vi "Load App.vi"(8 "error in (no error)":errorcluster) -> (0 "error out":errorcluster)   [LabVIEW 2013, in "LVAutomationListener.lvlib" / "LVAutomationListener.lvclass"]
doc: "Load the application into memory and start it running. The input notifier is used to send text to the splash screen to tell the user what stage the load process is in."
uses:
  LVAutomationListener.lvclass
  <vilib>/ActorFramework/Message Queue/Message Queue.lvclass/Message Queue.ctl
  <vilib>/Utility/error.llb/DialogType.ctl
  <vilib>/ActorFramework/Actor/Actor.lvclass
  <vilib>/ActorFramework/Message Queue/Message Queue.lvclass
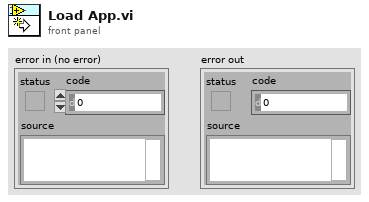
[diagram p1: front panel]
types:
  T1 = typedef "DialogType.ctl" = u16
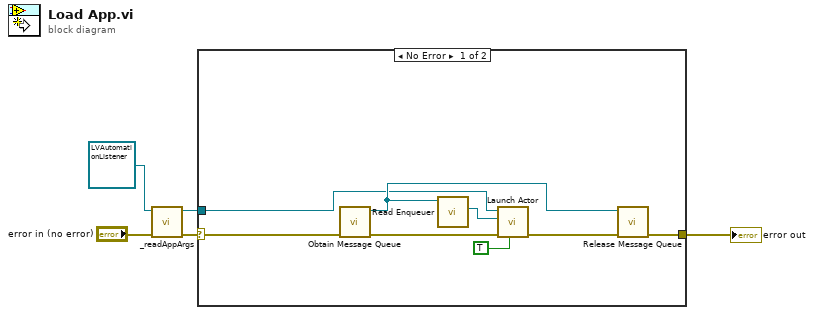
[diagram p0: block diagram]
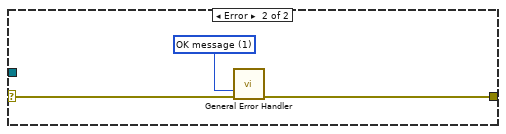
[diagram p2: hidden frame]
diagram:
  n1 = call "_readAppArgs.vi"("error in (no error)"="error in (no error)", "LVAutomationListener in"=refnum<class "LVAutomationListener.lvclass"> refnum ("My Application.lvclass")) -> ("error out"=w2:errorcluster, "LVAutomationListener out"=w1:refnum<class "LVAutomationListener.lvclass">)  [unwired: 8 in]
  n2 = case shown="No Error" w2 {
    selector: w2 -> [w6 w16]
    tunnel: w1 -> [w8 _]
    tunnel: [w7 w14] -> w3
    frame No Error {
      n3 = call <vilib>:"Obtain Message Queue.vi"("error in (no error)"=w6) -> ("error out"=w11:errorcluster, "Message Queue"=w10:refnum<class "Message Queue.lvclass">)  [unwired: 9 in]
      n4 = call <vilib>:"Read Enqueuer.vi"("Message Queue"=w10) -> ("Message Enqueuer"=w13:refnum<class "Message Enqueuer.lvclass">)  [unwired: 10 in]
      n5 = call <vilib>:"Launch Actor.vi"("Open Actor Core front panel? (F)"=TRUE, "error in (no error)"=w11, "Actor-to-Caller Enqueuer"=w13, "Actor"=w8) -> ("error out"=w12:errorcluster)  [unwired: 6 in, 1 out]
      n6 = call <vilib>:"Release Message Queue.vi"("error in (no error)"=w12, "Message Queue"=w10) -> ("error out"=w7:errorcluster)  [unwired: 8 in, 1 out]
    }
    frame Error {
      w15 = T1 1 items=["no dialog", "OK message", "continue or stop message", "OK message + warnings", "continue/stop + warnings"] ("type of dialog (OK msg:1)")
      n7 = call <vilib>:"General Error Handler.vi"("type of dialog (OK msg:1)"=w15, "error in (no error)"=w16) -> ("error out"=w14:errorcluster)  [unwired: 9 in, 4 out]
    }
  }
  "error out" <- w3
